vi "PathToLinuxPath.vi"(11 "Path in":path) -> (3 "Path out":path)   [LabVIEW 2016, in "Scan Engine Custom Device.lvlib"]
uses:
  Scan Engine Custom Device.lvlib
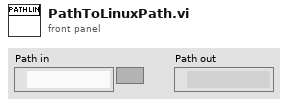
[diagram p1: front panel]
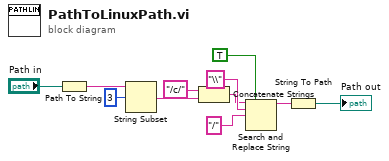
[diagram p0: block diagram]
diagram:
  n1 = Path To String(path="Path in") -> (string=w11:string)
  n2 = String Subset(string=w11, offset (0)=3) -> (substring=w2:string)  [unwired: 1 in]
  n3 = Concatenate Strings("/c/" ("string"), w2) -> (w3:string)
  n4 = Search and Replace String(replace all?=TRUE ("replace all? (F)"), input string=w3, search string="\\", replace string="/" ("replace string (\"\")")) -> (result string=w8:string)  [unwired: 4 in, 3 out]
  n5 = String To Path(string=w8) -> (path=→"Path out":path)
